vi "Read Motor Controller Constants.vi"(8 "error in (no error)":errorcluster, 10 "settings in":variant, 11 "Tank Drive in":refnum<class "Tank Drive.lvclass">) -> (0 "error out":errorcluster, 3 "Tank Drive out":refnum<class "Tank Drive.lvclass">)   [LabVIEW 2019, in "Drive.lvlib" / "Tank Drive.lvclass"]
uses:
  Tank Drive.lvclass
  00be1c54-a4dc-4847-a327-bb4ac6293fe5.vi
  <vilib>/Rock Robotics/WPI/ThirdParty/Phoenix-LabVIEW/Motor Controller/Controls/CTRE_Phoenix_MotorControl_SlotStructure.ctl
  DriveOld/Controls/Drive Sensor Data.ctl
  DriveOld/Drive.lvclass
  DriveOld/Controls/Motion Magic Constants.ctl
  Controls/Constants.ctl
  649c2bd3-2dcd-4980-bd27-aea9d7bf1900.vi
  8df500da-e1ee-44d6-a592-6dc076d38f0c.vi
  54dfd019-40a4-4691-a125-5d556ca44713.vi
  e599d267-a30b-413c-9052-4e958f4ba8d6.vi
  d68d9618-f3a8-403f-b0a1-099962ca1e3b.vi
  595c15e3-3b41-454f-8752-700bf276a686.vi
  56cca836-0b15-45fa-8748-7bd786a23e12.vi
  <vilib>/Rock Robotics/WPI/ThirdParty/Phoenix-LabVIEW/Motor Controller/Controls/CTRE_Phoenix_MotorControl_SupplyCurrentLimitConfiguration.ctl
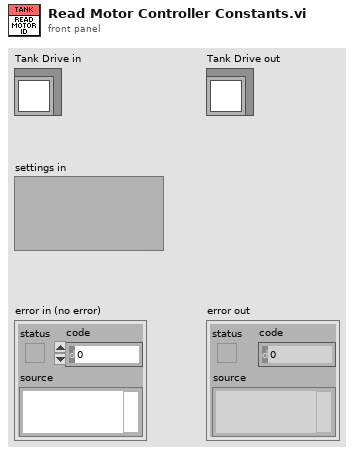
[diagram p1: front panel]
types:
  T1 = typedef "Drive.lvlib/Tank Drive.lvclass/Constants.ctl" = cluster{"Drive Velocity Low Gear":T2, "Drive Velocity High Gear":T2, "Drive Motion Magic Primary Low Gear":T2, "Drive Motion Magic Primary High Gear":T2, "Drive Motion Magic Secondary Low Gear":T2, "Drive Motion Magic Secondary High Gear":T2, "Drive Sensors":T3, "Motion Magic Constants":T4, "Supply Current Limit Configuration":T5}
  T2 = typedef "CTRE_Phoenix_MotorControl_SlotStructure.ctl" = cluster{"P":dbl, "I":dbl, "D":dbl, "F":dbl, "integralZone":dbl, "allowableClosedLoopError":i32, "maxIntegralAccumulator":dbl, "closedLoopPeakOutput":dbl, "closedLoopPeriod":i32}
  T3 = typedef "DriveOld.lvlib/Drive.lvclass/Drive Sensor Data.ctl" = cluster{"Drive Right Invert":bool, "Drive Right Sensor Phase":bool, "Drive Left Invert":bool, "Drive Left Sensor Phase":bool}
  T4 = typedef "DriveOld.lvlib/Drive.lvclass/Motion Magic Constants.ctl" = cluster{"Low Gear Max Velocity":u32, "High Gear Max Velocity":u32, "Motion Magic Low Gear Max Velocity":u32, "Motion Magic Low Gear Max Acceleration":u32, "Motion Magic High Gear Max Velocity":u32, "Motion Magic High Gear Max Acceleration":u32}
  T5 = typedef "CTRE_Phoenix_MotorControl_SupplyCurrentLimitConfiguration.ctl" = cluster{"Enable?":bool, "Current Limit":dbl, "Threshold Current":dbl, "Threshold Time":dbl}
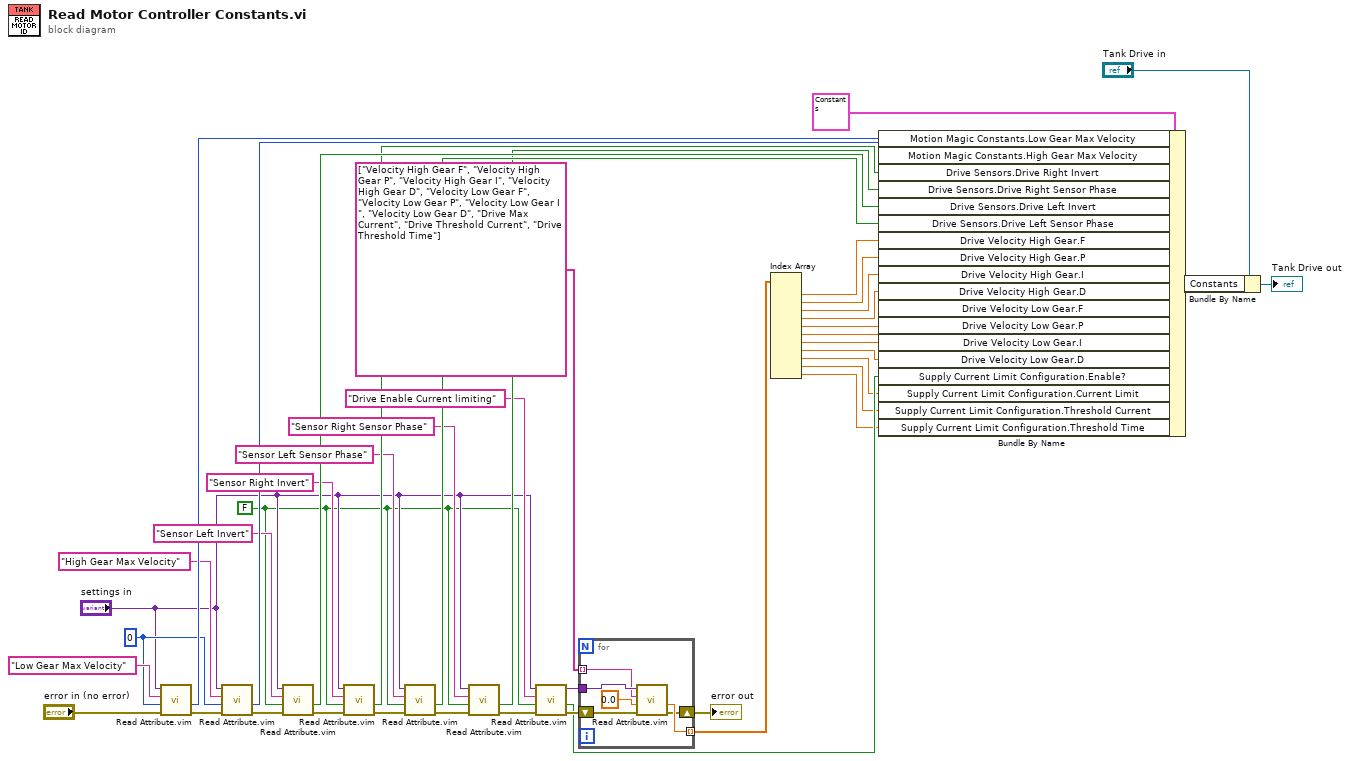
[diagram p0: block diagram]
diagram:
  w4 = FALSE
  w36 = 0
  n1 = call "Read Attribute.vim"("error in"="error in (no error)", "default value (data type)"=w36, "name"="Low Gear Max Velocity", "variant in"="settings in") -> ("error out"=w26:errorcluster, "value"=w38:i32)  [unwired: 4 in, 2 out]
  n2 = call "Read Attribute.vim"("error in"=w26, "default value (data type)"=w36, "name"="High Gear Max Velocity", "variant in"="settings in") -> ("error out"=w25:errorcluster, "value"=w35:i32)  [unwired: 4 in, 2 out]
  n3 = call "Read Attribute.vim"("error in"=w25, "default value (data type)"=w4, "name"="Sensor Left Invert", "variant in"="settings in") -> ("error out"=w24:errorcluster, "value"=w33:bool)  [unwired: 4 in, 2 out]
  n4 = call "Read Attribute.vim"("error in"=w24, "default value (data type)"=w4, "name"="Sensor Right Invert", "variant in"="settings in") -> ("error out"=w23:errorcluster, "value"=w31:bool)  [unwired: 4 in, 2 out]
  n5 = call "Read Attribute.vim"("error in"=w23, "default value (data type)"=w4, "name"="Sensor Left Sensor Phase", "variant in"="settings in") -> ("error out"=w22:errorcluster, "value"=w29:bool)  [unwired: 4 in, 2 out]
  n6 = call "Read Attribute.vim"("error in"=w22, "default value (data type)"=w4, "name"="Sensor Right Sensor Phase", "variant in"="settings in") -> ("error out"=w10:errorcluster, "value"=w27:bool)  [unwired: 4 in, 2 out]
  n7 = call "Read Attribute.vim"("error in"=w10, "default value (data type)"=w4, "name"="Drive Enable Current limiting", "variant in"="settings in") -> ("error out"=w9:errorcluster, "value"=w5:bool, "variant out"=w6:variant)  [unwired: 4 in, 1 out]
  n8 = for {
    tunnel: w6 -> [w50]
    tunnel: string[] ["Velocity High Gear F", "Velocity High Gear P", "Velocity High Gear I", "Velocity High Gear D", "Velocity Low Gear F", "Velocity Low Gear P", "Velocity Low Gear I ", "Velocity Low Gear D", "Drive Max Current", "Drive Threshold Current", "Drive Threshold Time"] -> [w49] mode=indexing
    tunnel: [w47] -> w19 mode=indexing
    shift-right: [w45] -> w20
    shift-left: w9 -> [w46]
    n9 = call "Read Attribute.vim"("error in"=w46, "default value (data type)"=0.0, "name"=w49, "variant in"=w50) -> ("error out"=w45:errorcluster, "value"=w47:dbl)  [unwired: 4 in, 2 out]
  }
  "error out" <- w20
  n10 = Index Array(array=w19) -> (element #1=w18:dbl, element #2=w17:dbl, element #3=w16:dbl, element #4=w15:dbl, element #5=w14:dbl, element #6=w13:dbl, element #7=w12:dbl, element #8=w11:dbl, element #9=w3:dbl, element #10=w2:dbl, element #11=w1:dbl)  [unwired: 11 in]
  n11 = Bundle By Name(cluster=T1 {"Drive Velocity Low Gear"={"P"=0.0, "I"=0.0, "D"=0.0, "F"=0.0, "integralZone"=0.0, "allowableClosedLoopError"=0, "maxIntegralAccumulator"=0.0, "closedLoopPeakOutput"=1.0, "closedLoopPeriod"=1}, "Drive Velocity High Gear"={"P"=0.0, "I"=0.0, "D"=0.0, "F"=0.0, "integralZone"=0.0, "allowableClosedLoopError"=0, "maxIntegralAccumulator"=0.0, "closedLoopPeakOutput"=1.0, "closedLoopPeriod"=1}, "Drive Motion Magic Primary Low Gear"={"P"=0.0, "I"=0.0, "D"=0.0, "F"=0.0, "integralZone"=0.0, "allowableClosedLoopError"=0, "maxIntegralAccumulator"=0.0, "closedLoopPeakOutput"=1.0, "closedLoopPeriod"=1}, "Drive Motion Magic Primary High Gear"={"P"=0.0, "I"=0.0, "D"=0.0, "F"=0.0, "integralZone"=0.0, "allowableClosedLoopError"=0, "maxIntegralAccumulator"=0.0, "closedLoopPeakOutput"=1.0, "closedLoopPeriod"=1}, "Drive Motion Magic Secondary Low Gear"={"P"=0.0, "I"=0.0, "D"=0.0, "F"=0.0, "integralZone"=0.0, "allowableClosedLoopError"=0, "maxIntegralAccumulator"=0.0, "closedLoopPeakOutput"=1.0, "closedLoopPeriod"=1}, "Drive Motion Magic Secondary High Gear"={"P"=0.0, "I"=0.0, "D"=0.0, "F"=0.0, "integralZone"=0.0, "allowableClosedLoopError"=0, "maxIntegralAccumulator"=0.0, "closedLoopPeakOutput"=1.0, "closedLoopPeriod"=1}, "Drive Sensors"={"Drive Right Invert"=FALSE, "Drive Right Sensor Phase"=FALSE, "Drive Left Invert"=FALSE, "Drive Left Sensor Phase"=FALSE}, "Motion Magic Constants"={"Low Gear Max Velocity"=20000, "High Gear Max Velocity"=40000, "Motion Magic Low Gear Max Velocity"=20000, "Motion Magic Low Gear Max Acceleration"=10000, "Motion Magic High Gear Max Velocity"=40000, "Motion Magic High Gear Max Acceleration"=20000}, "Supply Current Limit Configuration"={"Enable?"=FALSE, "Current Limit"=0.0, "Threshold Current"=0.0, "Threshold Time"=0.0}} ("Constants"), "Motion Magic Constants.Low Gear Max Velocity"=w38, "Motion Magic Constants.High Gear Max Velocity"=w35, "Drive Sensors.Drive Right Invert"=w31, "Drive Sensors.Drive Right Sensor Phase"=w27, "Drive Sensors.Drive Left Invert"=w33, "Drive Sensors.Drive Left Sensor Phase"=w29, "Drive Velocity High Gear.F"=w18, "Drive Velocity High Gear.P"=w17, "Drive Velocity High Gear.I"=w16, "Drive Velocity High Gear.D"=w15, "Drive Velocity Low Gear.F"=w14, "Drive Velocity Low Gear.P"=w13, "Drive Velocity Low Gear.I"=w12, "Drive Velocity Low Gear.D"=w11, "Supply Current Limit Configuration.Enable?"=w5, "Supply Current Limit Configuration.Current Limit"=w3, "Supply Current Limit Configuration.Threshold Current"=w2, "Supply Current Limit Configuration.Threshold Time"=w1) -> (w39:T1)
  n12 = Bundle By Name(cluster="Tank Drive in", "Constants"=w39) -> (→"Tank Drive out":refnum<class "Tank Drive.lvclass">)
